vi "UDP_in.vi"(3 "data in":string, 8 "error in (no error)":errorcluster, 9 "Panelka port":u16, 10 "Env port":u16) -> (0 "error out":errorcluster, 2 "data out":string)   [LabVIEW 2019]
panel:
  in  "Enviroment IP":string
  out "size(s)":i32
  out "My IP 2":string
  out "My IP":string
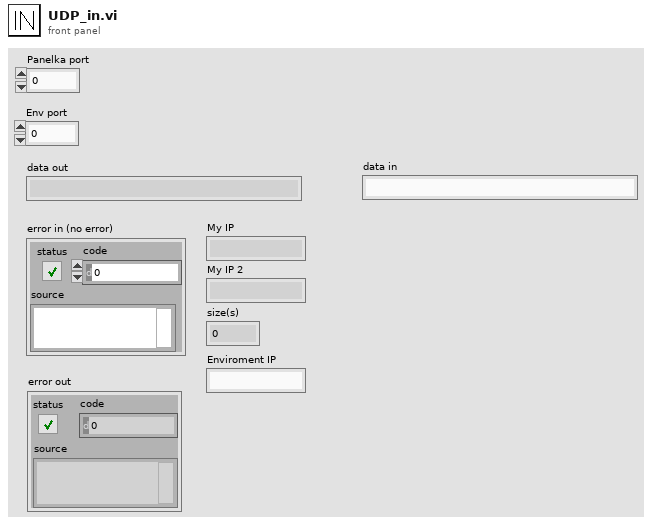
[diagram p1: front panel]
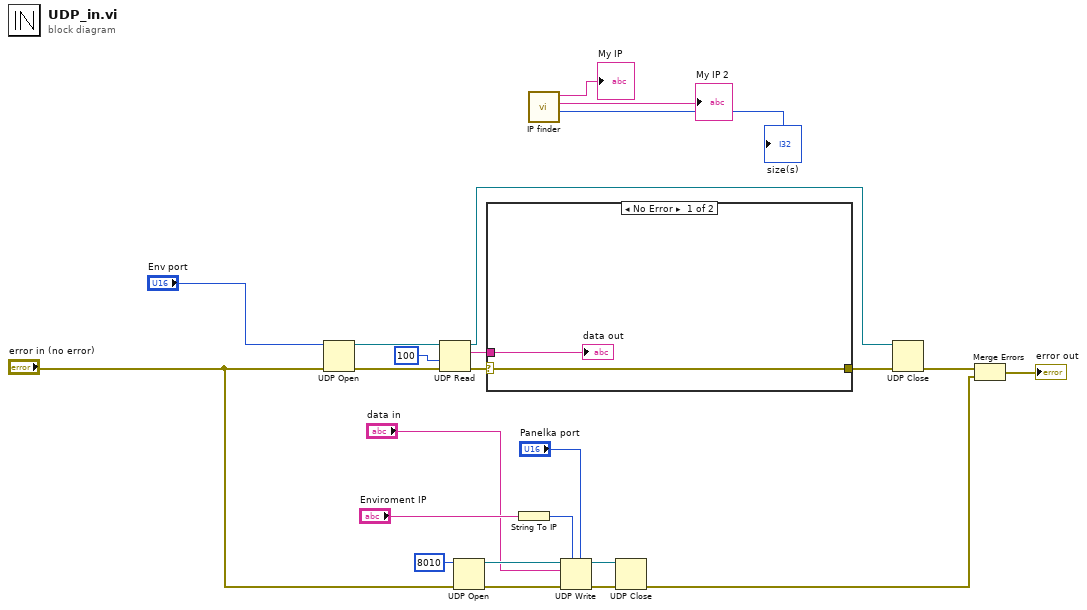
[diagram p0: block diagram]
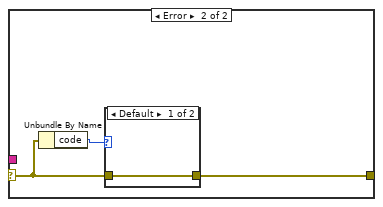
[diagram p2: hidden frame]
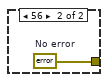
[diagram p3: hidden frame]
diagram:
  n1 = UDP Open(8:"error in (no error)", 11:"Env port") -> (port=w23:refnum<k16>, 0:w22:errorcluster)  [unwired: 3 in, 1 out]
  n2 = UDP Read(connection ID=w23, timeout ms (25000)=100, 8:w22) -> (data out=w19:string, error out=w20:errorcluster, 3:w18:refnum<k16>)  [unwired: 1 in, 2 out]
  n3 = UDP Open(8:"error in (no error)", 11:u16 8010 ("port")) -> (port=w7:refnum<k16>, 0:w8:errorcluster)  [unwired: 3 in, 1 out]
  n4 = case shown="No Error" w20 {
    selector: w20 -> [w26 w28]
    tunnel: [w26 w27] -> w17
    tunnel: w19 -> [w25 _]
    frame No Error {
      "data out" <- w25
    }
    frame Error {
      # "Sender did not send data. Ignore timeout error and keep waiting."
      n5 = Unbundle By Name(w28) -> ("code"=w29:i32)
      n6 = case shown="Default" w29 {
        tunnel: w28 -> [w30 _]
        tunnel: [w30 w31] -> w27
        frame Default {
        }
        frame 56 {
          w31 = errorcluster {"status"=FALSE, "code"=0, "source"=""}  # No error
        }
      }
    }
  }
  n7 = String To IP(1:"Enviroment IP") -> (0:w11:u32)
  n8 = call "IP finder.vi"() -> ("size(s)"=→"size(s)":i32, "My IP 2"=→"My IP 2":string, "My IP"=→"My IP":string)  [unwired: 9 in]
  n9 = UDP Write(address=w11, port or service name="Panelka port", connection ID=w7, data in="data in", 8:w8) -> (error out=w9:errorcluster, 3:w10:refnum<k16>)  [unwired: 1 in]
  n10 = UDP Close(connection ID=w10, 8:w9) -> (error out=w1:errorcluster)  [unwired: 1 out]
  n11 = UDP Close(connection ID=w18, 8:w17) -> (error out=w3:errorcluster)  [unwired: 1 out]
  n12 = Merge Errors(w3, w1) -> (→"error out":errorcluster)
